vi "Desktop Execution - Generate Test Data.vi"() -> (3 "Random Number":dbl min=-1.7976931348623157e+308 max=1.7976931348623157e+308)   [LabVIEW 2023]
doc: "This VI generates random number and output it to <B>Generate User-Defined Trace Event</B>."
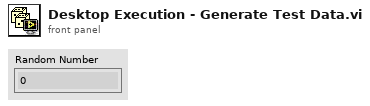
[diagram p1: front panel]
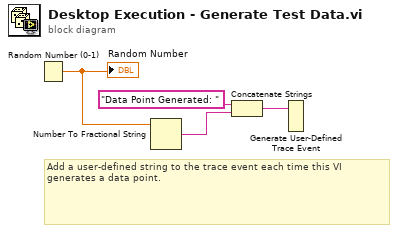
[diagram p0: block diagram]
diagram:
  # "Add a user-defined string to the trace event each time this VI generates a data point."
  n1 = Random Number (0-1)() -> (number: 0 to 1=w4:dbl)
  "Random Number" <- w4
  n2 = Number To Fractional String(number=w4) -> (F-format string=w2:string)  [unwired: 3 in]
  n3 = Concatenate Strings("Data Point Generated: " ("string"), w2) -> (w1:string)
  n4 = Generate User-Defined Trace Event(2:w1) -> ()  [unwired: 1 out]
